vi "OpenSerial.vi"(8 "error in (no error)":errorcluster, 11 "properties":T1[](array[typedef])) -> (0 "error out":errorcluster, 1 "read timeout (ms)":i32, 2 "read interval (sec)":dbl, 3 "serial master instance":refnum<class "Modbus Master.lvclass">)   [LabVIEW 2017, in "ModbusMaster.lvlib"]
uses:
  <vilib>/addons/InsightCM/Devices/Shared/Common/ModbusMaster/ModbusMaster.lvlib
  <vilib>/Modbus/master/Modbus Master.lvclass
  <vilib>/addons/InsightCM/MessageBus/Base/controls/KeyValuePair.ctl
  <vilib>/Modbus/master/Create Master Instance (Serial).vi
  <vilib>/addons/InsightCM/Utilities/PropertyHelpers/PropertyHelpers.lvlib
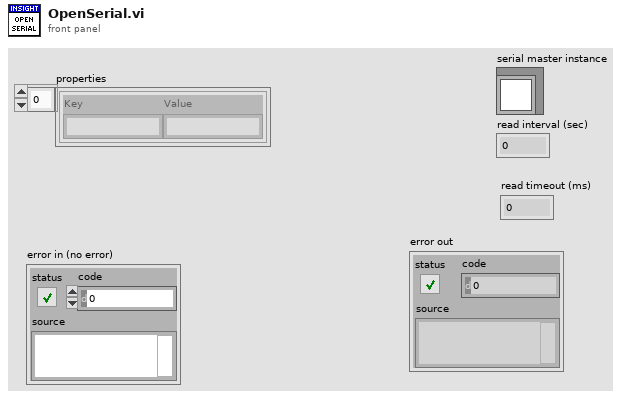
[diagram p1: front panel]
types:
  T1 = typedef "KeyValuePair.ctl" = cluster{"Key":string, "Value":string}
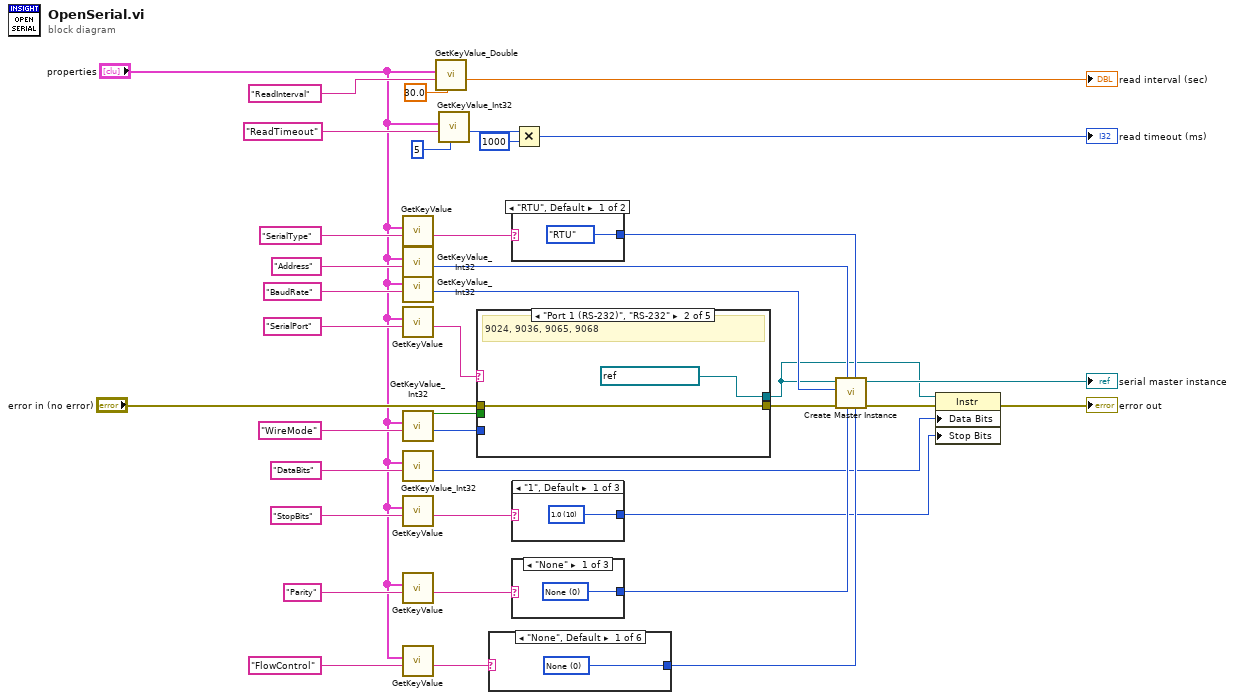
[diagram p0: block diagram]
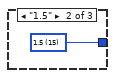
[diagram p2: hidden frame]
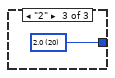
[diagram p3: hidden frame]
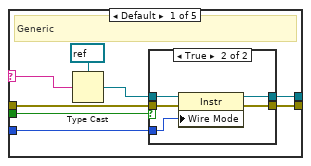
[diagram p4: hidden frame]
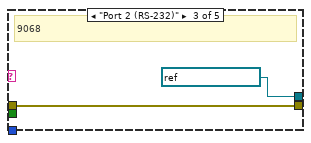
[diagram p6: hidden frame]
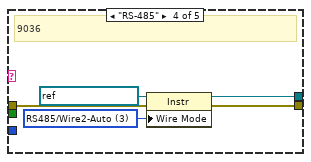
[diagram p7: hidden frame]
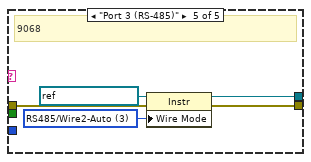
[diagram p8: hidden frame]
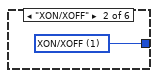
[diagram p9: hidden frame]
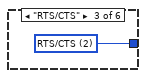
[diagram p10: hidden frame]
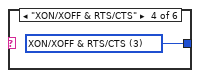
[diagram p11: hidden frame]
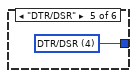
[diagram p12: hidden frame]
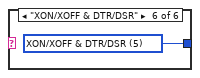
[diagram p13: hidden frame]
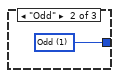
[diagram p14: hidden frame]
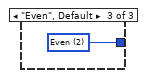
[diagram p15: hidden frame]
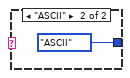
[diagram p16: hidden frame]
diagram:
  n1 = call <vilib>:"GetKeyValue.vi"("key"="SerialType", "key value pairs"="properties") -> ("value"=w36:string)  [unwired: 7 in, 2 out]
  n2 = call <vilib>:"GetKeyValue_Int32.vi"("key"="Address", "key value pairs"="properties") -> ("value"=w33:i32)  [unwired: 7 in, 2 out]
  n3 = call <vilib>:"GetKeyValue_Int32.vi"("key"="BaudRate", "key value pairs"="properties") -> ("value"=w30:i32)  [unwired: 7 in, 2 out]
  n4 = call <vilib>:"GetKeyValue.vi"("key"="SerialPort", "key value pairs"="properties") -> ("value"=w19:string)  [unwired: 7 in, 2 out]
  n5 = call <vilib>:"GetKeyValue_Int32.vi"("key"="WireMode", "key value pairs"="properties") -> ("value"=w8:i32, "found"=w7:bool)  [unwired: 7 in, 1 out]
  n6 = call <vilib>:"GetKeyValue_Int32.vi"("key"="DataBits", "key value pairs"="properties") -> ("value"=w12:i32)  [unwired: 7 in, 2 out]
  n7 = call <vilib>:"GetKeyValue.vi"("key"="StopBits", "key value pairs"="properties") -> ("value"=w11:string)  [unwired: 7 in, 2 out]
  n8 = call <vilib>:"GetKeyValue.vi"("key"="Parity", "key value pairs"="properties") -> ("value"=w29:string)  [unwired: 7 in, 2 out]
  n9 = call <vilib>:"GetKeyValue.vi"("key"="FlowControl", "key value pairs"="properties") -> ("value"=w26:string)  [unwired: 7 in, 2 out]
  n10 = call <vilib>:"GetKeyValue_Double.vi"("default"=30.0, "key"="ReadInterval", "key value pairs"="properties") -> ("value"=→"read interval (sec)":dbl)  [unwired: 6 in, 2 out]
  n11 = call <vilib>:"GetKeyValue_Int32.vi"("default"=5, "key"="ReadTimeout", "key value pairs"="properties") -> ("value"=w4:i32)  [unwired: 6 in, 2 out]
  n12 = case shown="\"Port 1 (RS-232)\", \"RS-232\"" w19 {
    selector: w19 -> [w42 _ _ _ _]
    tunnel: "error in (no error)" -> [w46 w54 w56 w60 w65]
    tunnel: [w45 refnum<visa-resource-name> "ASRL1::INSTR" ("VISA resource name") refnum<visa-resource-name> "ASRL2::INSTR" ("VISA resource name") w59 w64] -> w15
    tunnel: [w44 w54 w56 w58 w63] -> w17
    tunnel: w8 -> [w39 _ _ _ _]
    tunnel: w7 -> [w40 _ _ _ _]
    frame Default {
      # "Generic"
      n13 = Type Cast(type=refnum<visa-resource-name> refnum ("reference"), x=w42) -> (*(type *) &x=w41:refnum<visa-resource-name>)
      n14 = case shown="True" w40 {
        tunnel: w46 -> [w47 w53]
        tunnel: [w48 w52] -> w45
        tunnel: [w47 w51] -> w44
        tunnel: w41 -> [w48 w50]
        tunnel: w39 -> [_ w49]
        frame False {
        }
        frame True {
          n15 = property class="Instr"(reference=w50, error in=w53, "Wire Mode"=w49) -> (reference out=w52:refnum<visa-resource-name>, error out=w51:errorcluster)
        }
      }
    }
    frame "Port 1 (RS-232)", "RS-232" {
      # "9024, 9036, 9065, 9068"
    }
    frame "Port 2 (RS-232)" {
      # "9068"
    }
    frame "RS-485" {
      w61 = i16 3 items=["Unknown"=-1, "RS485/Wire4"=0, "RS485/Wire2-EchoDTR"=1, "RS485/Wire2-CtrlDTR"=2, "RS485/Wire2-Auto"=3, "RS232/DTE"=128, "RS232/DCE"=129, "RS232/AUTO"=130] ("Serial Settings:Wire Mode")
      # "9036"
      n16 = property class="Instr"(reference=refnum<visa-resource-name> "ASRL2::INSTR" ("VISA resource name"), error in=w60, "Wire Mode"=w61) -> (reference out=w59:refnum<visa-resource-name>, error out=w58:errorcluster)
    }
    frame "Port 3 (RS-485)" {
      w66 = i16 3 items=["Unknown"=-1, "RS485/Wire4"=0, "RS485/Wire2-EchoDTR"=1, "RS485/Wire2-CtrlDTR"=2, "RS485/Wire2-Auto"=3, "RS232/DTE"=128, "RS232/DCE"=129, "RS232/AUTO"=130] ("Serial Settings:Wire Mode")
      # "9068"
      n17 = property class="Instr"(reference=refnum<visa-resource-name> "ASRL3::INSTR" ("VISA resource name"), error in=w65, "Wire Mode"=w66) -> (reference out=w64:refnum<visa-resource-name>, error out=w63:errorcluster)
    }
  }
  n18 = case shown="\"None\", Default" w26 {
    tunnel: [w68 w69 w70 w71 w72 w73] -> w24
    frame "None", Default {
      w68 = u16 0 items=["None", "XON/XOFF", "RTS/CTS", "XON/XOFF & RTS/CTS", "DTR/DSR", "XON/XOFF & DTR/DSR"] ("flow control (None)")
    }
    frame "XON/XOFF" {
      w69 = u16 1 items=["None", "XON/XOFF", "RTS/CTS", "XON/XOFF & RTS/CTS", "DTR/DSR", "XON/XOFF & DTR/DSR"] ("flow control (None)")
    }
    frame "RTS/CTS" {
      w70 = u16 2 items=["None", "XON/XOFF", "RTS/CTS", "XON/XOFF & RTS/CTS", "DTR/DSR", "XON/XOFF & DTR/DSR"] ("flow control (None)")
    }
    frame "XON/XOFF & RTS/CTS" {
      w71 = u16 3 items=["None", "XON/XOFF", "RTS/CTS", "XON/XOFF & RTS/CTS", "DTR/DSR", "XON/XOFF & DTR/DSR"] ("flow control (None)")
    }
    frame "DTR/DSR" {
      w72 = u16 4 items=["None", "XON/XOFF", "RTS/CTS", "XON/XOFF & RTS/CTS", "DTR/DSR", "XON/XOFF & DTR/DSR"] ("flow control (None)")
    }
    frame "XON/XOFF & DTR/DSR" {
      w73 = u16 5 items=["None", "XON/XOFF", "RTS/CTS", "XON/XOFF & RTS/CTS", "DTR/DSR", "XON/XOFF & DTR/DSR"] ("flow control (None)")
    }
  }
  n19 = case shown="\"RTU\", Default" w36 {
    tunnel: [enum16{"RTU", "ASCII"}."RTU" ("serial type") enum16{"RTU", "ASCII"}."ASCII" ("serial type")] -> w35
    frame "RTU", Default {
    }
    frame "ASCII" {
    }
  }
  n20 = case shown="\"1\", Default" w11 {
    tunnel: [w76 w77 w78] -> w10
    frame "1", Default {
      w76 = u16 10 items=["1.0"=10, "1.5"=15, "2.0"=20] ("Serial Settings:Stop Bits")
    }
    frame "1.5" {
      w77 = u16 15 items=["1.0"=10, "1.5"=15, "2.0"=20] ("Serial Settings:Stop Bits")
    }
    frame "2" {
      w78 = u16 20 items=["1.0"=10, "1.5"=15, "2.0"=20] ("Serial Settings:Stop Bits")
    }
  }
  n21 = case shown="\"None\"" w29 {
    tunnel: [w79 w80 w81] -> w25
    frame "None" {
      w79 = u16 0 items=["None", "Odd", "Even"] ("parity (Even)")
    }
    frame "Odd" {
      w80 = u16 1 items=["None", "Odd", "Even"] ("parity (Even)")
    }
    frame "Even", Default {
      w81 = u16 2 items=["None", "Odd", "Even"] ("parity (Even)")
    }
  }
  n22 = Multiply(x=w4, y=1000) -> (x*y=→"read timeout (ms)":i32)
  n23 = call-poly <vilib>:"Create Master Instance.vi"("flow control (None)"=w24, "serial type"=w35, "parity (Even)"=w25, "unit ID"=w33, "error in (no error)"=w17, "baud rate (9600)"=w30, "VISA resource name"=w15) -> ("error out"=w16:errorcluster, "serial master instance"=→"serial master instance":refnum<class "Modbus Master.lvclass">)  [unwired: 3 in]
  n24 = property class="Instr"(reference=w15, error in=w16, "Data Bits"=w12, "Stop Bits"=w10) -> (error out=→"error out":errorcluster)  [unwired: 1 out]
